vi "Workspace Tool with Event Messages.vi"() -> ()   [LabVIEW 2016]
uses:
  NationalInstruments.VeriStand.SystemStorageUI
  NationalInstruments.VeriStand.SystemStorage
  <vilib>/NI Veristand/Templates/Workspace Tool Support/Workspace Tool Message Bus.ctl
  <vilib>/NI Veristand/Templates/Workspace Tool Support/Workspace Tool Message (String).ctl
  <vilib>/NI Veristand/Templates/Workspace Tool Support/Workspace Tool Response (String).ctl
  <vilib>/NI Veristand/Templates/Workspace Tool Support/Workspace Tool Message (Byte Array).ctl
  <vilib>/NI Veristand/Templates/Workspace Tool Support/Workspace Tool Response (Byte Array).ctl
  <vilib>/NI Veristand/Execution/Workspace/NI VeriStand - Get Multiple Channel Values.vi
  <vilib>/NI VeriStand/Execution/Workspace/NI_VS Workspace ExecutionAPI.lvlib
  <vilib>/NI Veristand/UI Controls/Single Node Browser/NI_VS UI Single Node Browser.lvlib
  <vilib>/NI VeriStand/Templates/Workspace Tool Support/NI VeriStand - Workspace Tool Support.lvlib
panel:
  in  "NIVS.Message Bus":T1
  out "Byte Array Data":u8[](array[numeric])
  out "String Data":string
  in  "Stop":bool
  in  "NIVS.System Definition Root":refnum<k24>
  in  "Tree Browser":refnum<k24>(container)
  in  "NIVS.Project File Path":path
  in  "Single Node Browser":refnum<k24>(container)
  in  "NIVS.Workspace Event":refnum<event-registration>
  out "System Times":dbl[](array[numeric]) format="%<%H:%M:%S%3u>t"
  out "Targets":string[](array[string])
  in  "NIVS.Gateway IP Address":string
  in  "NIVS.INI File Path":path
  # "Use this example as a template to create custom tools for the NI VeriStand Workspace. This example shows the use of the NI VeriStand API and UI controls to set and get data.\n\nRun this example by adding this VI as a Workspace Tool item. For Help adding Workspace Tool items, please reference the NI VeriStand Help."
  # "This code is used to register events from the\nNI VeriStand - Send Workspace Tool Message VI"
  # "With the assistance of the NI VeriStand Execution API, a tool has access to streaming data running on the target."
  # "This is the file path to the VeriStand system definition file. You can read or write to the file using the System Definition API."
  # "This is the root reference to the active System Definition file. You could use this to read the configuration or populate a tree with channels. You are free to close this reference, but it will be closed for you if you don't."
  # "The SystemStorageUI .NET assembly provides controls to display data configured in the System Definition file."
  # "This is the IP Address of the VeriStand Gateway to which the Workspace is connected. Use this to open all the .NET Manager references. Usually the Gateway is running on localhost, but it could be running on a neighbor's machine."
  # "This registered string User Event is used to help instruct your tool to shut down when the Workspace is closing."
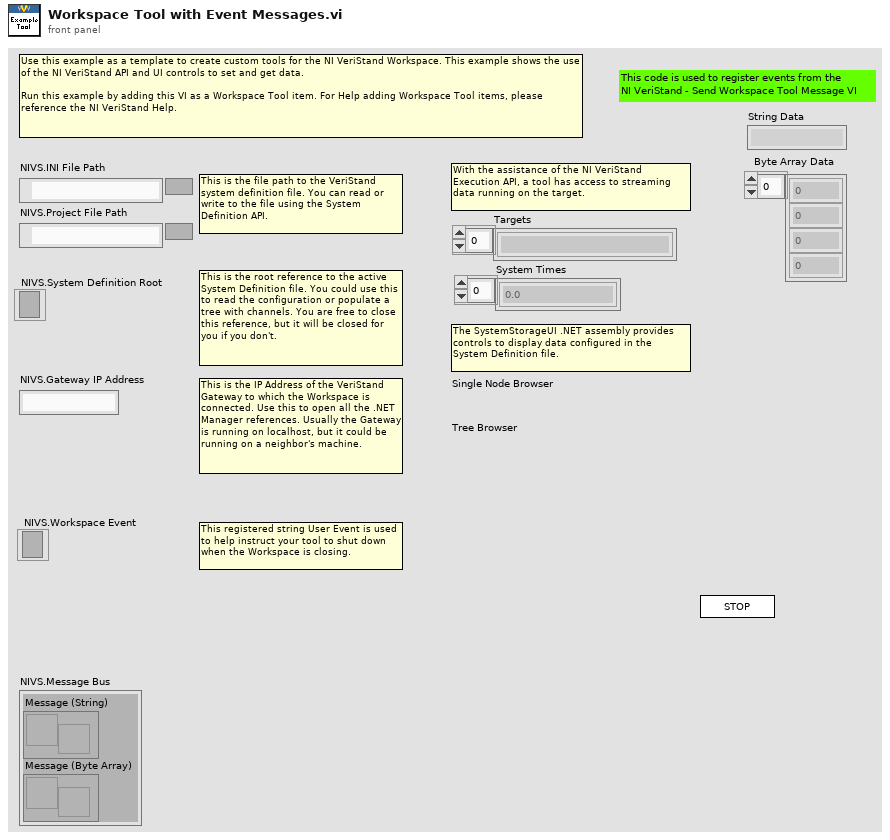
[diagram p1: front panel]
types:
  T1 = typedef "NI VeriStand - Workspace Tool Support.lvlib/Workspace Tool Message Bus.ctl" = cluster{"Message (String)":refnum<user-event>, "Message (Byte Array)":refnum<user-event>}
  T2 = typedef "NI_VS UI Single Node Browser.lvlib/Callback Type.ctl" = cluster{"Net Callbacks":refnum<k27>[], "Event":refnum<user-event>}
  T3 = typedef "NI_VS Workspace ExecutionAPI.lvlib/WorkspaceAPI.ctl" = refnum<k24>
  T4 = typedef "NI_VS Workspace ExecutionAPI.lvlib/SystemStateEventRef.ctl" = cluster{"CustDatRef":refnum<user-event>, "EvtRef":refnum<k27>, "Target State User Event":refnum<user-event>}
  T5 = typedef "NI_VS Workspace ExecutionAPI.lvlib/SystemStateRegEventRef.ctl" = refnum<event-registration>
  T6 = cluster{"NIVS.Workspace Event":refnum<event-registration>, "Event Registration Refnum":refnum<event-registration>, "Event Registration Refnum":refnum<event-registration>, "SystemChangeEventRef":T5}
  T7 = typedef "NI_VS UI Single Node Browser.lvlib/Node Ref.ctl" = refnum<k24>
  T8 = typedef "NI VeriStand - Workspace Tool Support.lvlib/Workspace Tool Response (String).ctl" = cluster{"Response":string, "Error":errorcluster}
  T9 = typedef "NI VeriStand - Workspace Tool Support.lvlib/Workspace Tool Response (Byte Array).ctl" = cluster{"Response":u8[], "Error":errorcluster}
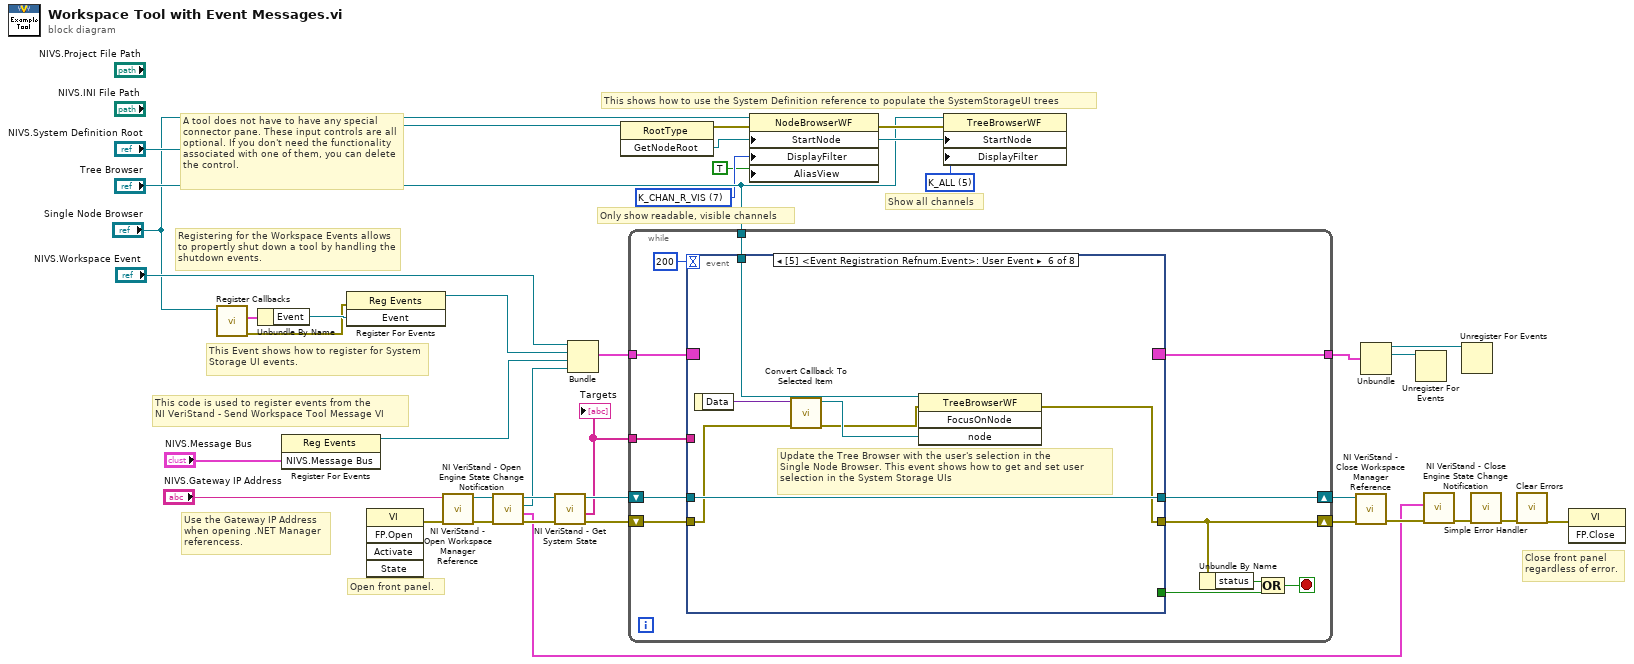
[diagram p0: block diagram]
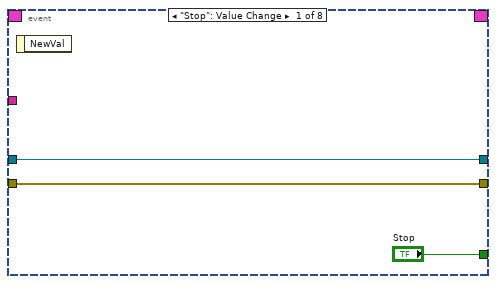
[diagram p2: hidden frame]
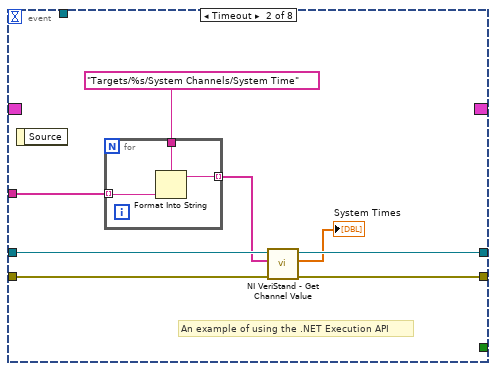
[diagram p3: hidden frame]
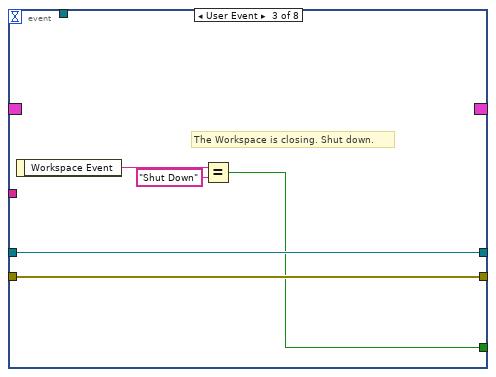
[diagram p4: hidden frame]
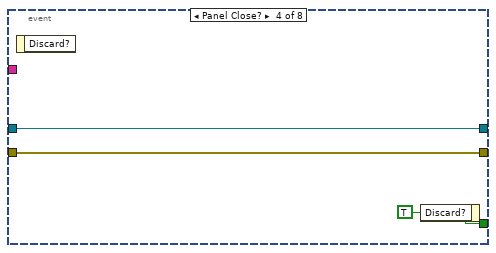
[diagram p5: hidden frame]
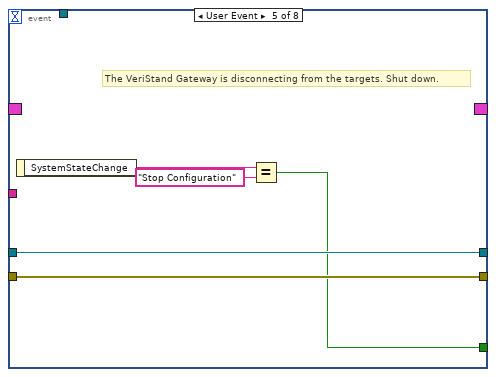
[diagram p6: hidden frame]
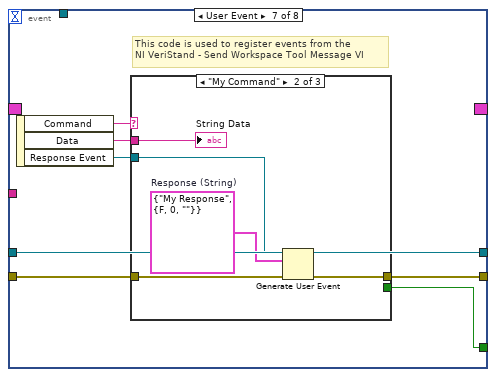
[diagram p7: hidden frame]
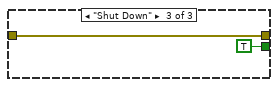
[diagram p9: hidden frame]
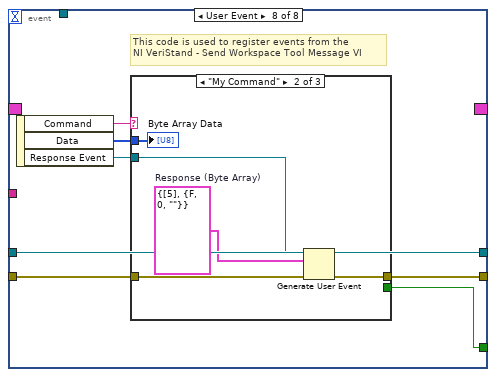
[diagram p10: hidden frame]
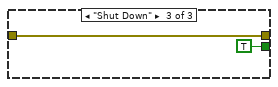
[diagram p12: hidden frame]
diagram:
  w9 = u8 7 items=["K_CHAN_R", "K_CHAN_W", "K_CHAN_RW", "K_CHAN_VOLT", "K_CHAN_FAULT", "K_ALL", "K_CUSTOM", "K_CHAN_R_VIS", "K_CHAN_W_VIS", "K_CHAN_RW_VIS", "K_CHAN_VOLT_VIS", "K_CHAN_FAULT_VIS"] ("DisplayFilter")
  w10 = u8 5 items=["K_CHAN_R", "K_CHAN_W", "K_CHAN_RW", "K_CHAN_VOLT", "K_CHAN_FAULT", "K_ALL", "K_CUSTOM", "K_CHAN_R_VIS", "K_CHAN_W_VIS", "K_CHAN_RW_VIS", "K_CHAN_VOLT_VIS", "K_CHAN_FAULT_VIS"] ("DisplayFilter")
  # "This code is used to register events from the\nNI VeriStand - Send Workspace Tool Message VI"
  # "Show all channels"
  # "Only show readable, visible channels"
  # "This Event shows how to register for System Storage UI events."
  # "Use the Gateway IP Address when opening .NET Manager referencess."
  # "A tool does not have to have any special connector pane. These input controls are all optional. If you don't need the functionality associated with one of them, you can delete the control."
  # "This shows how to use the System Definition reference to populate the SystemStorageUI trees"
  # "Registering for the Workspace Events allows to propertly shut down a tool by handling the shutdown events."
  # "Close front panel\nregardless of error."
  # "Open front panel."
  n1 = call <vilib>:"Register Callbacks.vi"("Single Node Browser"="Single Node Browser") -> ("error out"=w4:errorcluster, "Callbacks"=w6:T2)  [unwired: 8 in, 1 out]
  n2 = Unbundle By Name(w6) -> ("Event"=w5:refnum<user-event>)
  n3 = register-events("NIVS.Message Bus") -> (reference out=w1:refnum<event-registration>)  [unwired: 2 in, 1 out]
  n4 = register-events(error in=w4, w5) -> (reference out=w12:refnum<event-registration>)  [unwired: 1 in, 1 out]
  n5 = invoke class="VI" method="FP.Open"() -> (error out=w20:errorcluster)  [unwired: 5 in, 4 out]
  n6 = call <vilib>:"NI VeriStand - Open Workspace Manager Reference.vi"("error in (no error)"=w20, "Gateway IP Address (\"\": localhost)"="NIVS.Gateway IP Address") -> ("error out"=w31:errorcluster, "WorkspaceManager"=w32:T3)  [unwired: 8 in]
  n7 = call <vilib>:"NI VeriStand - Open Engine State Change Notification.vi"("error in (no error)"=w31, "WorkspaceManager in"=w32) -> ("error out"=w36:errorcluster, "SystemStateRefs"=w25:T4, "SystemChangeEventRef"=w2:T5, "WorkspaceManager out"=w37:T3)  [unwired: 6 in]
  n8 = call <vilib>:"NI VeriStand - Get System State.vi"("error in (no error)"=w36, "WorkspaceManager in"=w37) -> ("error out"=w23:errorcluster, "Targets"=w22:string[], "WorkspaceManager  out"=w24:T3)  [unwired: 5 in, 2 out]
  "Targets" <- w22
  n9 = Bundle("NIVS.Workspace Event"="NIVS.Workspace Event", "Event Registration Refnum"=w12, "Event Registration Refnum"=w1, "SystemChangeEventRef"=w2) -> (w30:T6)  [unwired: 1 in]
  n10 = invoke class="RootType" method="GetNodeRoot"(reference="NIVS.System Definition Root") -> (error out=w14:errorcluster, "GetNodeRoot"=w15:refnum<k24>)  [unwired: 2 in, 1 out]
  n11 = while {
    tunnel: w30 -> [w49]
    tunnel: [w48] -> w29
    shift-right: [w41] -> w33
    shift-left: w23 -> [w46]
    shift-right: [w45] -> w34
    shift-left: w24 -> [w47]
    tunnel: w22 -> [w43]
    tunnel: "Tree Browser" -> [w38]
    stop <- w39 stop-if-true
    n12 = event shown="[5] <Event Registration Refnum.Event>: User Event" {
      selector: w49 -> [_ _ _ _ _ _ _ _]
      dyn-events: [_ _ _ _ _ _ _ _] -> w48
      timeout: 200 -> [_ _ _ _ _ _ _ _]
      tunnel: ["Stop" _ w64 w69 w72 _ w87 w102] -> w40
      tunnel: w47 -> [w51 w60 w67 w70 w75 w83 w90 w105]
      tunnel: w46 -> [w52 w59 w68 w71 w76 w79 w89 w104]
      tunnel: [w52 w54 w68 w71 w76 w77 w86 w101] -> w41
      tunnel: [w51 w55 w67 w70 w75 w83 w90 w105] -> w45
      tunnel: w43 -> [_ w58 _ _ _ _ _ _]
      tunnel: w38 -> [_ _ _ _ _ w82 _ _]
      event "Stop": Value Change {
        n13 = event-data() -> ()  [unwired: 1 in, 1 out]
      }
      event Timeout {
        # "An example of using the .NET Execution API"
        n14 = event-data() -> ()  [unwired: 1 in, 1 out]
        n15 = for {
          tunnel: w58 -> [w62] mode=indexing
          tunnel: "Targets/%s/System Channels/System Time" ("format string") -> [w63]
          tunnel: [w61] -> w56 mode=indexing
          n16 = Format Into String(format string=w63, w62) -> (resulting string=w61:string)  [unwired: 2 in, 1 out]
        }
        n17 = call-poly <vilib>:"NI VeriStand - Get Channel Value.vi"("error in (no error)"=w59, "Channels"=w56, "WorkspaceManager in"=w60) -> ("error out"=w54:errorcluster, "Values"=→"System Times":dbl[], "WorkspaceManager out"=w55:T3)  [unwired: 6 in]
      }
      event User Event {
        # "The Workspace is closing. Shut down."
        n18 = event-data() -> ("Workspace Event"=w66:string)  [unwired: 1 in]
        n19 = Equal?(x=w66, y="Shut Down") -> (x = y?=w64:bool)
      }
      event Panel Close? {
        w69 = TRUE ("Discard?")
        n20 = event-data() -> ()  [unwired: 1 in, 1 out]
        n21 = event-data("Discard?"=w69) -> ()  [unwired: 1 in, 1 out]
      }
      event User Event {
        # "The VeriStand Gateway is disconnecting from the targets. Shut down."
        n22 = event-data() -> ("SystemStateChange"=w74:string)  [unwired: 1 in]
        n23 = Equal?(x=w74, y="Stop Configuration") -> (x = y?=w72:bool)
      }
      event User Event {
        # "Update the Tree Browser with the user's selection in the\nSingle Node Browser. This event shows how to get and set user\nselection in the System Storage UIs"
        n24 = event-data() -> ("Data"=w81:variant)  [unwired: 1 in]
        n25 = call <vilib>:"Convert Callback To Selected Item.vi"("error in"=w79, "Data"=w81) -> ("error out"=w78:errorcluster, "Selected Item"=w80:T7)  [unwired: 8 in]
        n26 = invoke class="TreeBrowserWF" method="FocusOnNode"(reference=w82, error in=w78, "node"=w80) -> (error out=w77:errorcluster)  [unwired: 1 in, 3 out]
      }
      event User Event {
        # "This code is used to register events from the\nNI VeriStand - Send Workspace Tool Message VI"
        n27 = event-data() -> ("Command"=w88:string, "Data"=w85:string, "Response Event"=w84:refnum<user-event>)  [unwired: 1 in]
        n28 = case shown="\"My Command\"" w88 {
          tunnel: w89 -> [w91 w95 w97]
          tunnel: [_ _ TRUE] -> w87
          tunnel: [w91 w94 w97] -> w86
          tunnel: w85 -> [_ w93 _]
          tunnel: w84 -> [_ w92 _]
          frame Default {
          }
          frame "My Command" {
            w96 = T8 {"Response"="My Response", "Error"={"status"=FALSE, "code"=0, "source"=""}}  # Response (String)
            n29 = Generate User Event(user event=w92, event data cluster=w96, error in=w95) -> (error out=w94:errorcluster)  [unwired: 1 in, 1 out]
            "String Data" <- w93
          }
          frame "Shut Down" {
          }
        }
      }
      event User Event {
        # "This code is used to register events from the\nNI VeriStand - Send Workspace Tool Message VI"
        n30 = event-data() -> ("Command"=w103:string, "Data"=w100:u8[], "Response Event"=w99:refnum<user-event>)  [unwired: 1 in]
        n31 = case shown="\"My Command\"" w103 {
          tunnel: w104 -> [w106 w111 w112]
          tunnel: [_ _ TRUE] -> w102
          tunnel: [w106 w110 w112] -> w101
          tunnel: w100 -> [_ w108 _]
          tunnel: w99 -> [_ w109 _]
          frame Default {
          }
          frame "My Command" {
            w107 = T9 {"Response"=[5], "Error"={"status"=FALSE, "code"=0, "source"=""}}  # Response (Byte Array)
            n32 = Generate User Event(user event=w109, event data cluster=w107, error in=w111) -> (error out=w110:errorcluster)  [unwired: 1 in, 1 out]
            "Byte Array Data" <- w108
          }
          frame "Shut Down" {
          }
        }
      }
    }
    n33 = Unbundle By Name(w41) -> ("status"=w42:bool)
    n34 = Compound Arithmetic op=OR(w42, w40) -> (w39:bool)
  }
  n35 = property class="NodeBrowserWF"(reference="Single Node Browser", error in=w14, "StartNode"=w15, "DisplayFilter"=w9, "AliasView"=TRUE) -> (error out=w16:errorcluster)  [unwired: 1 out]
  n36 = property class="TreeBrowserWF"(reference="Tree Browser", error in=w16, "StartNode"=w15, "DisplayFilter"=w10) -> ()  [unwired: 2 out]
  n37 = call <vilib>:"NI VeriStand - Close Workspace Manager Reference.vi"("error in (no error)"=w33, "WorkspaceManager"=w34) -> ("error out"=w26:errorcluster)  [unwired: 9 in]
  n38 = Unbundle(w29) -> ("NIVS.Workspace Event"=w27:refnum<event-registration>, "Event Registration Refnum"=w28:refnum<event-registration>)  [unwired: 2 out]
  n39 = Unregister For Events(event registration refnum=w28) -> ()  [unwired: 1 in, 1 out]
  n40 = call <vilib>:"NI VeriStand - Close Engine State Change Notification.vi"("error in (no error)"=w26, "SystemStateRefs"=w25) -> ("error out"=w19:errorcluster)  [unwired: 9 in]
  n41 = Unregister For Events(event registration refnum=w27) -> ()  [unwired: 1 in, 1 out]
  n42 = call <vilib>:"Simple Error Handler.vi"("error in (no error)"=w19) -> ("error out"=w18:errorcluster)  [unwired: 4 in, 4 out]
  n43 = call <vilib>:"Clear Errors.vi"("error in (no error)"=w18) -> ("error out"=w17:errorcluster)  [unwired: 5 in, 1 out]
  n44 = invoke class="VI" method="FP.Close"(error in=w17) -> ()  [unwired: 2 in, 3 out]
